vi "MAINRIJDEN.vi"() -> ()   [LabVIEW 2018]
doc: "Use this template to build a standard state machine design pattern. Each state executes code and determines which state to transition to. Contrast this design pattern with the User Interface Event Handler pattern, in which code executes in response to user actions. Contrast this design pattern also with the Queued Message Handler pattern, in which each message handling code can queue zero or more new messages."
uses:
  FSM States.ctl
panel:
  out "Motor":bool[](array[boolean])
  out "Current state":T1
  in  "Blokje gepakt":bool
  in  "Eindloopschakelaar":bool
  in  "Afstandssensor":i32
  in  "Start vooruit":bool
  in  "ON/OFF":bool
  # "Stopt programma als uit is"
  # "Afstand in centimeter"
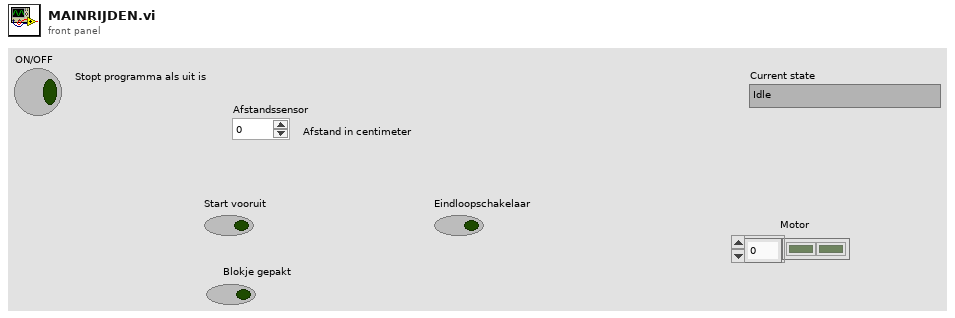
[diagram p1: front panel]
types:
  T1 = typedef "FSM States.ctl" = enum16{"Idle", "Vooruit", "Achteruit"}
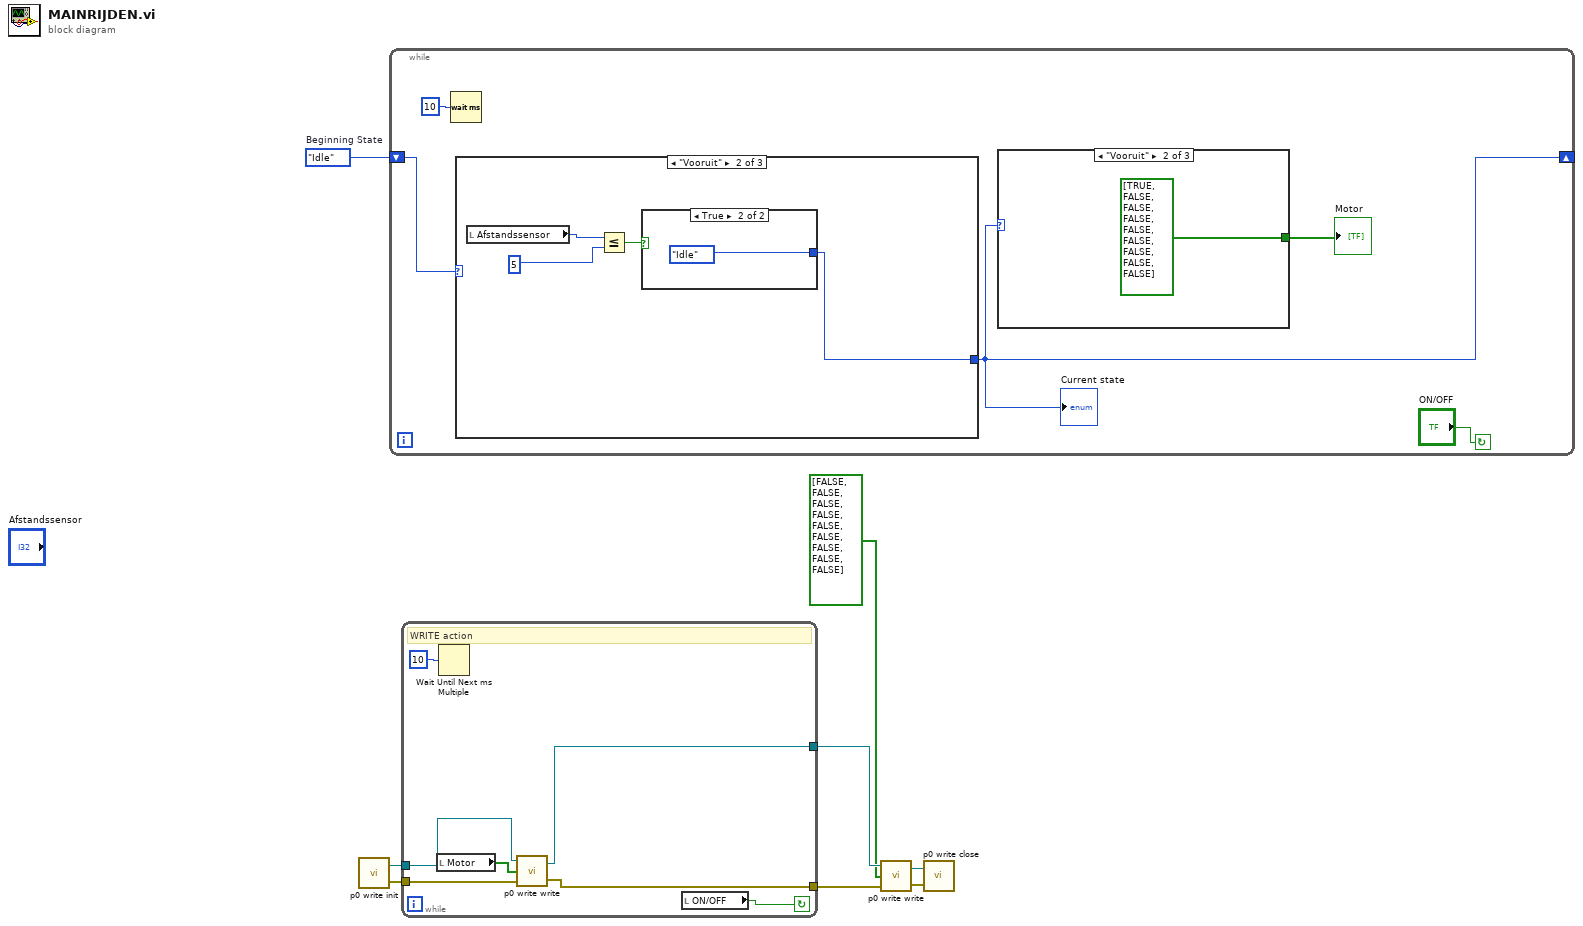
[diagram p0: block diagram]
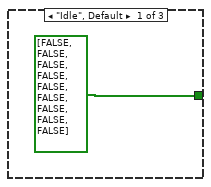
[diagram p2: hidden frame]
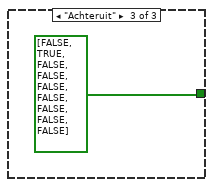
[diagram p3: hidden frame]
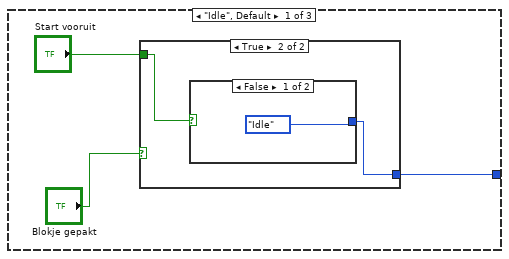
[diagram p4: hidden frame]
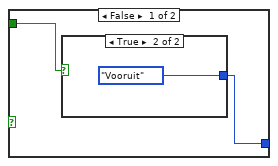
[diagram p5: hidden frame]
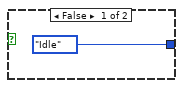
[diagram p6: hidden frame]
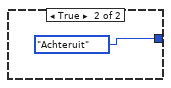
[diagram p7: hidden frame]
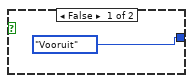
[diagram p8: hidden frame]
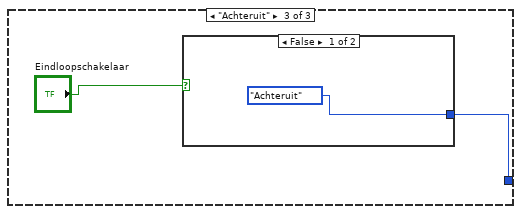
[diagram p9: hidden frame]
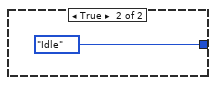
[diagram p10: hidden frame]
diagram:
  w8 = FSM_States."Idle"  # Beginning State
  n1 = call "p0 write init.vi"() -> ("error out"=w2:errorcluster, "task out"=w3:refnum<k21>)
  n2 = while {
    shift-right: [w10] -> _
    shift-left: w8 -> [w13]
    stop <- "ON/OFF" continue-if-true
    n3 = Wait (ms)(milliseconds to wait=u32 10) -> ()  [unwired: 1 out]
    n4 = case shown="\"Vooruit\"" w13 {
      tunnel: [w18 w31 w34] -> w10
      frame "Idle", Default {
        n5 = case shown="True" "Blokje gepakt" {
          tunnel: "Start vooruit" -> [w21 w25]
          tunnel: [w20 w24] -> w18
          frame False {
            n6 = case shown="True" w21 {
              tunnel: [FSM_States."Idle" FSM_States."Vooruit"] -> w20
              frame False {
              }
              frame True {
              }
            }
          }
          frame True {
            n7 = case shown="False" w25 {
              tunnel: [FSM_States."Idle" FSM_States."Achteruit"] -> w24
              frame False {
              }
              frame True {
              }
            }
          }
        }
      }
      frame "Vooruit" {
        n8 = local read "Afstandssensor"() -> (w30:i32)
        n9 = Less Or Equal?(x=w30, y=5) -> (x <= y?=w29:bool)
        n10 = case shown="True" w29 {
          tunnel: [FSM_States."Vooruit" FSM_States."Idle"] -> w31
          frame False {
          }
          frame True {
          }
        }
      }
      frame "Achteruit" {
        n11 = case shown="False" "Eindloopschakelaar" {
          tunnel: [FSM_States."Achteruit" FSM_States."Idle"] -> w34
          frame False {
          }
          frame True {
          }
        }
      }
    }
    "Current state" <- w10
    n12 = case shown="\"Vooruit\"" w10 {
      tunnel: [bool[] [FALSE, FALSE, FALSE, FALSE, FALSE, FALSE, FALSE, FALSE, FALSE] ("digital out") bool[] [TRUE, FALSE, FALSE, FALSE, FALSE, FALSE, FALSE, FALSE, FALSE] ("digital out") bool[] [FALSE, TRUE, FALSE, FALSE, FALSE, FALSE, FALSE, FALSE, FALSE] ("digital out")] -> w9
      frame "Idle", Default {
      }
      frame "Vooruit" {
      }
      frame "Achteruit" {
      }
    }
    "Motor" <- w9
  }
  n13 = while {
    tunnel: w3 -> [w44]
    tunnel: [w43] -> w7
    tunnel: w2 -> [w42]
    tunnel: [w40] -> w6
    stop <- w39 continue-if-true
    # "WRITE action"
    n14 = local read "Motor"() -> (w38:bool[])
    n15 = Wait Until Next ms Multiple(millisecond multiple=u32 10) -> ()  [unwired: 1 out]
    n16 = call "p0 write write.vi"("error in"=w42, "digital out"=w38, "task/channels in"=w44) -> ("error out"=w40:errorcluster, "task out"=w43:refnum<k21>)
    n17 = local read "ON/OFF"() -> (w39:bool)
  }
  n18 = call "p0 write write.vi"("error in"=w6, "digital out"=bool[] [FALSE, FALSE, FALSE, FALSE, FALSE, FALSE, FALSE, FALSE, FALSE], "task/channels in"=w7) -> ("error out"=w4:errorcluster, "task out"=w5:refnum<k21>)
  n19 = call "p0 write close.vi"("error in"=w4, "task/channels in"=w5) -> ()
